vi "Keyence.Main-Init.vi"(7 "Idx":i32, 8 "error in":errorcluster, 10 "restart (T)":bool=TRUE) -> (0 "error out":errorcluster)   [LabVIEW 2015]
uses:
  Keyence.Action.ctl
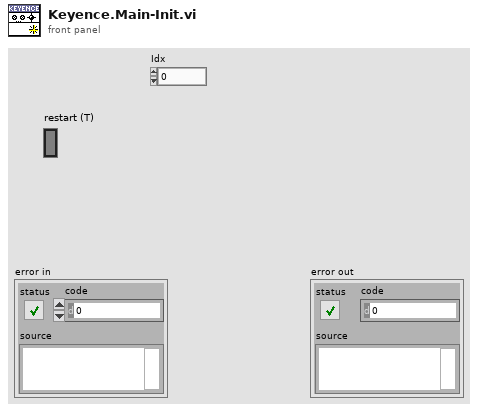
[diagram p1: front panel]
types:
  T1 = typedef "Keyence.Action.ctl" = enum32{"idle", "constructor", "destructor", "--- Keyence ---", "Init", "Scan"}
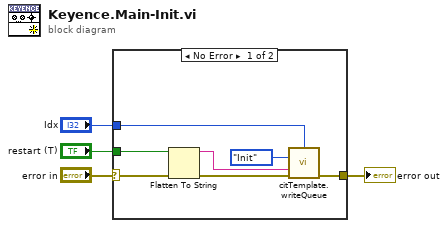
[diagram p0: block diagram]
diagram:
  n1 = case shown="No Error" "error in" {
    selector: "error in" -> [w11 w12]
    tunnel: [w9 w12] -> w3
    tunnel: "Idx" -> [w8 _]
    tunnel: "restart (T)" -> [w6 _]
    frame No Error {
      n2 = Flatten To String(anything=w6, error in (no error)=w11) -> (data string=w5:string, error out=w7:errorcluster)  [unwired: 2 in, 1 out]
      n3 = call "citTemplate.writeQueue.vi"("instance (0)"=w8, "event in (if not connected:all statemachine with data event)"=Keyence.Action."Init" ("Action"), "data in"=w5, "error in (no error)"=w7) -> ("error out"=w9:errorcluster)  [unwired: 11 in]
    }
    frame Error {
    }
  }
  "error out" <- w3
